vi "Dialog Boxes.vi"   [LabVIEW 2020]
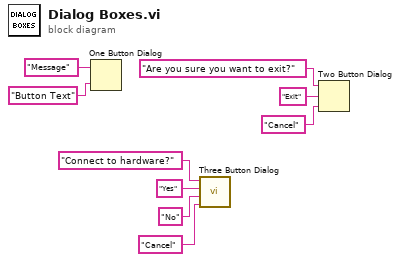
[diagram p0: block diagram]
diagram:
  n1 = One Button Dialog(message="Message", button name ("OK")="Button Text") -> ()  [unwired: 1 out]
  n2 = call <vilib>:"Three Button Dialog.vi"("Right Button Text (\"Cancel\")"="Cancel" ("Right Button Text (\"Cancel\")"), "Center Button Text (\"No\")"="No" ("Center Button Text (\"No\")"), "Left Button Text (\"Yes\")"="Yes" ("Left Button Text (\"Yes\")"), "message"="Connect to hardware?") -> ()  [unwired: 7 in, 1 out]
  n3 = Two Button Dialog(message="Are you sure you want to exit?", 1:"Cancel" ("F button name (\"Cancel\")"), 2:"Exit" ("T button name (\"OK\")")) -> ()  [unwired: 1 out]
